vi "ContrastAgent.vi"() -> ()   [LabVIEW 2022 SP3]
uses:
  ViewData/-ReadEye/Header.ctl
  <vilib>/Analysis/5stat.llb/RMS (DBL).vi
  <vilib>/Utility/file.llb/Write Delimited Spreadsheet (string).vi
  <vilib>/Analysis/NI_AALBase.lvlib
  <vilib>/Analysis/NI_AALPro.lvlib
panel:
  in  "Save data":bool
  in  "Header Out":T1={"header info"={"Header"="", "Head length"=0}, "A/D info"={"# rf points per line"=0, "# lines per scan"=0, "sample rate MHz"=0, "# A/D bits"=0, "# bytes per A/D"=0, "TGC Flag"=0, "A/D Type"=""}, "Tranducer Info"={"bandwidth"=0.0, "center freq"=0.0, "start freq"=0.0, "ID"=0}, "Scan Info"={"delay"=0.0, "pivot distance"=0.0, "sector scan angle"=0.0, "operator"="", "Scan Mode"="", "location"=""}, "Time/Date Info"={"date"="", "time"=""}, "RF Info"={"RF file name"="", "RF file att"="", "RF cal file name"="", "RF cal file att"=""}, "Patient Info"={"ID"="", "extended ID"="", "age"=0, "sex"="", "previously\nscanned"="", "PSA"=0.0, "LOS"=1, "Ethnicty 2"=3, "Race"=3}, "Tissue Type"={"organ"=0, "disease type"=0, "disease location"=0, "IQ_pts"=0, "RcvBuffer"=0, "RcvFrame"=0, "IQBuff"=0, "IQFrame"=0, "IQPage"=0}, "Votage scaling"={"Digitizer (dB)"=0.0, "Gain (dB)"=0.0, "Atten (dB)"=0.0}, "Comment"="", "Misc Info"={"avg num"=0, "c speed"=0, "Div By or SF zones"=0, "XMIT CHS"=0, "RCV CHS"=0, "Xmit angle"=0.0}, "Therapy Parameters"={"Theraputic Freq (MHz)"=0.0, "Time on (s)"=0.0, "Therapy amplitude (mV)"=0.0, "Lines Before"=0, "Lines After"=0}, "Scan Settings"={"Energy (uJ or V)"=0, "Damp (Ohm) or Fc"=0, "HP Filt (KHz)"=0, "LP Filt (MHz)"=0, "Gain (db)"=0, "prf (kHz)"=0.0, "Distance between\nscan lines (um)"=0, "Distance between\nscan planes (um)"=0, "Scan line gap (um)"=0.0, "Scan plane gap (um)"=0.0}, "Compression Parameters"={"F1 (MHz)"=0.0, "F2 (MHz)"=0.0, "% taper"=0.0, "duration"=0.0}, "Patient Info Xtra"={"First Name"="", "Last Name"="", "Notes"=""}, "ROI Box"=[0, 0, 0, 0]} {"Compression Parameters"."% taper" min=50 max=1000 format="%.2f"; "Compression Parameters"."F2 (MHz)" format="%.3f"; "Compression Parameters"."F1 (MHz)" format="%.3f"; "Scan Settings"."prf (kHz)" format="%.2f"; "Therapy Parameters"."Therapy amplitude (mV)" min=50 max=1000 format="%.2f"; "Therapy Parameters"."Time on (s)" format="%.3f"; "Therapy Parameters"."Theraputic Freq (MHz)" format="%.3f"; "Patient Info"."Race" items=["Am Ind or Alaska", "Asian", "Hawaiian, Pac Isl", "Black or Afr Amer", "White", "more than one race", "unknown"]; "Patient Info"."Ethnicty 2" items=["Hispanic", "Non-Hispanic", "unknown"]; "Patient Info"."LOS" items=["1", "2", "3", "4", "5"]; "Patient Info"."PSA" format="%.1f"; "Scan Info"."delay" format="%.2f"; "Scan Info"."pivot distance" format="%.2f"; "Scan Info"."sector scan angle" format="%.2f"; "Tranducer Info"."bandwidth" format="%.2f"; "Tranducer Info"."center freq" format="%.2f"; "Tranducer Info"."start freq" format="%.2f"}
  out "match substring":string
  out "noise level":dbl
  out "All Files":string[](array[string])
  out "agent in zone?":bool[](array[boolean])
  out "Array data to save":string[][](array[string])
  out "Numeric":i32
  out "average":sgl[][](array[numeric])
  out "Cts versus start line":i16[](graph)
  in  "How Many":i32
  in  "Sweep":bool
  out "Current file":string
  in  "Use Selected Files":bool
  in  "File Select":i32[](listbox)
  in  "Choose Top":path=path "\\\\vantage-n-wk\\Vantage Data/Adam Doppler/2016-08-12/HFR_03A_20D_08kHz_16MHz_00_EYE"
  in  "image to display":i32 min=0
  in  "start":i32
  out "Total Files":i32
  in  "# of files":i32=2000
  in  "Tab Control":enum32{"Contrast", "Variables"}(tab)
  out "Max dB each image":dbl[](graph)
  out "RF line":dbl[](graph)
  out "Velocity v time 2":dbl[](graph)
  out "Velocity v time":dbl[](graph)
  out "Binary Event Tracking":i16[](graph)
  out "First line":dbl[][](graph)
  out "Raw subset":dbl[][](graph)
  in  "start line":i32=10
  out "Raw data":dbl[][](graph)
  in  "Save  data":bool
  in  "RF Pt start":i32=100
  in  "RF Pts":i32=50
  in  "# rows":i32=17
  out "# drops":i32
  out "RMS noise":T2(graph)
  in  "RMS intervals":i32=10
  out "RMS Noise":dbl
  out "Correlation Shifts":T2(graph)
  in  "Corre Intervals":i32=10
  out "Max Local dB (absolute)":T2(graph)
  in  "Screening":T3={"dB Thresh"=-20.0, "Mask Start"=4, "Mask length"=3}
  out "max dB all":sgl
  out "Velocity":T2(graph)
  in  "Max dB intervals":i32=10
  in  "Vel Intevals":i32=10
  in  "Sub Average":bool
  in  "left rank":i32=2
  in  "dB Threshold":dbl=25.0
  in  "Simple Thresh Count?":bool
  out "Agent?":bool
  in  "fix RMS":dbl format="%0.2f"
  out "# in zone":i16
  in  "fix RMS?":bool
  out "Raw Complex output array":sgl[][][](array[numeric])
  out "Array":sgl[][](array[numeric])
  in  "read?":bool=TRUE
  in  "stop":bool
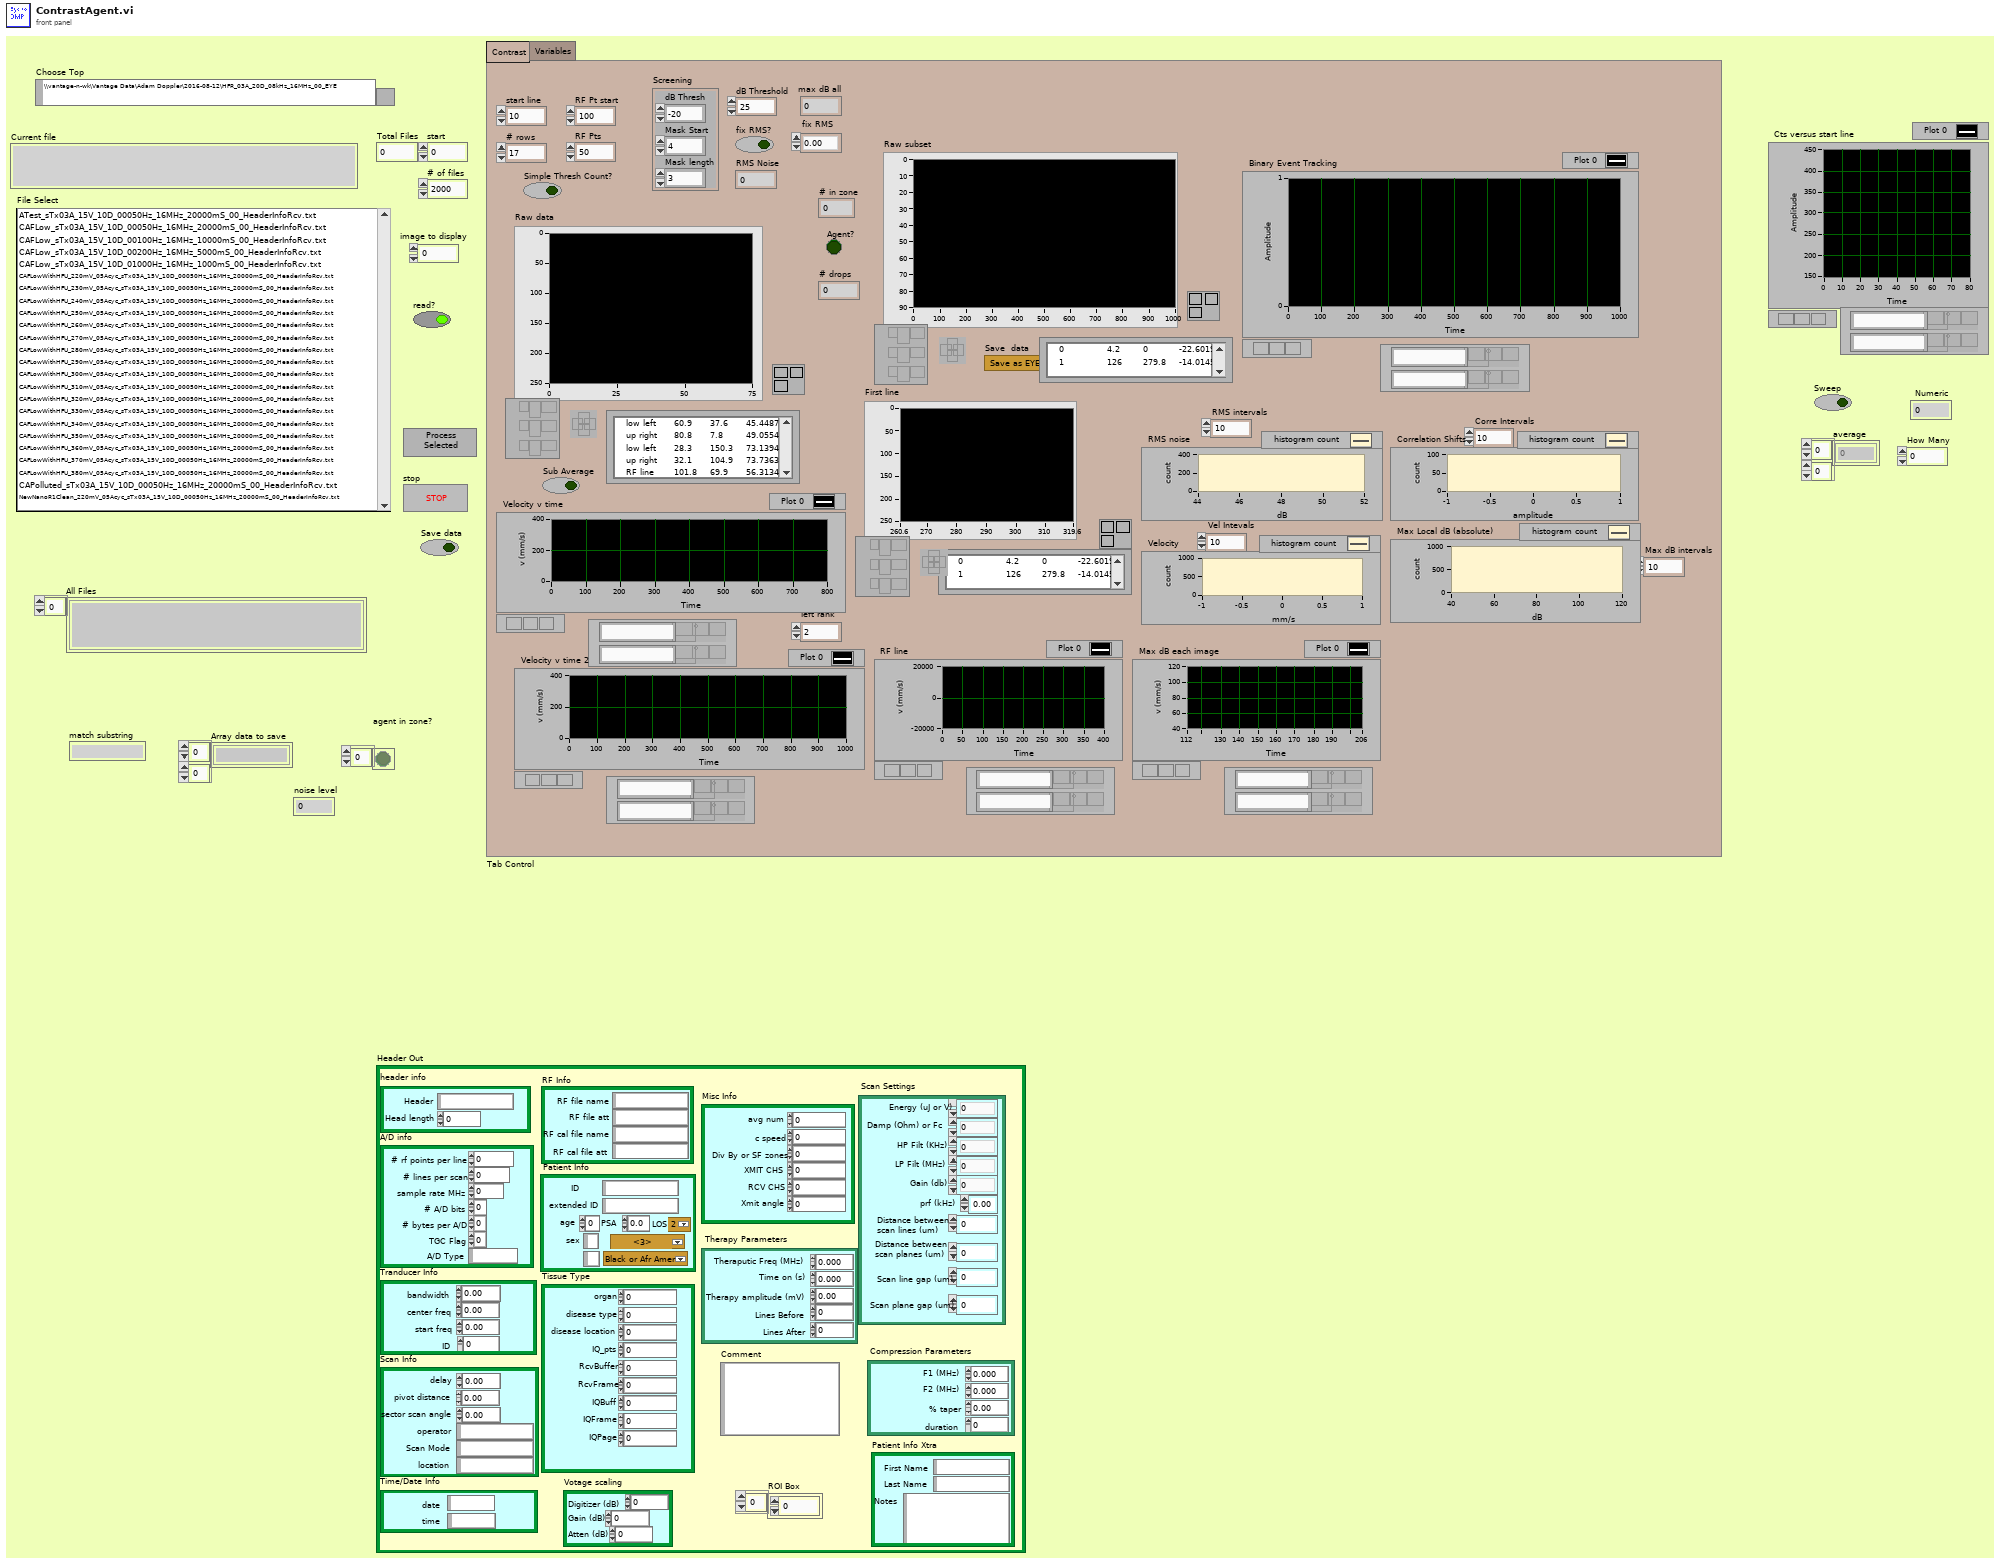
[diagram p1: front panel]
types:
  T1 = typedef "Header.ctl" = cluster{"header info":cluster{"Header":string, "Head length":i16}, "A/D info":cluster{"# rf points per line":u16, "# lines per scan":u16, "sample rate MHz":u16, "# A/D bits":i16, "# bytes per A/D":u16, "TGC Flag":u16, "A/D Type":string}, "Tranducer Info":cluster{"bandwidth":sgl, "center freq":sgl, "start freq":sgl, "ID":i32}, "Scan Info":cluster{"delay":sgl, "pivot distance":sgl, "sector scan angle":sgl, "operator":string, "Scan Mode":string, "location":string}, "Time/Date Info":cluster{"date":string, "time":string}, "RF Info":cluster{"RF file name":string, "RF file att":string, "RF cal file name":string, "RF cal file att":string}, "Patient Info":cluster{"ID":string, "extended ID":string, "age":u16, "sex":string, "previously\nscanned":string, "PSA":sgl, "LOS":u8, "Ethnicty 2":u8, "Race":u8}, "Tissue Type":cluster{"organ":i16, "disease type":i16, "disease location":i16, "IQ_pts":u16, "RcvBuffer":u8, "RcvFrame":u16, "IQBuff":u8, "IQFrame":u16, "IQPage":u8}, "Votage scaling":cluster{"Digitizer (dB)":sgl, "Gain (dB)":sgl, "Atten (dB)":sgl}, "Comment":string, "Misc Info":cluster{"avg num":u16, "c speed":i16, "Div By or SF zones":i16, "XMIT CHS":u8, "RCV CHS":u8, "Xmit angle":sgl}, "Therapy Parameters":cluster{"Theraputic Freq (MHz)":sgl, "Time on (s)":sgl, "Therapy amplitude (mV)":sgl, "Lines Before":u16, "Lines After":u16}, "Scan Settings":cluster{"Energy (uJ or V)":u8, "Damp (Ohm) or Fc":u8, "HP Filt (KHz)":u8, "LP Filt (MHz)":u8, "Gain (db)":u8, "prf (kHz)":sgl, "Distance between\nscan lines (um)":u16, "Distance between\nscan planes (um)":u16, "Scan line gap (um)":sgl, "Scan plane gap (um)":sgl}, "Compression Parameters":cluster{"F1 (MHz)":sgl, "F2 (MHz)":sgl, "% taper":sgl, "duration":sgl}, "Patient Info Xtra":cluster{"First Name":string, "Last Name":string, "Notes":string}, "ROI Box":u16[]}
  T2 = cluster{"X Values":dbl[], "Histogram: h(x)":i32[]}
  T3 = cluster{"dB Thresh":dbl, "Mask Start":i32, "Mask length":i32}
  T4 = enum16{"None", "Raw RF + time stamp", "Save IQAll", "Save IQSum", "Save IQSumReal", "Save Img", "Time Stamps", "unused"}
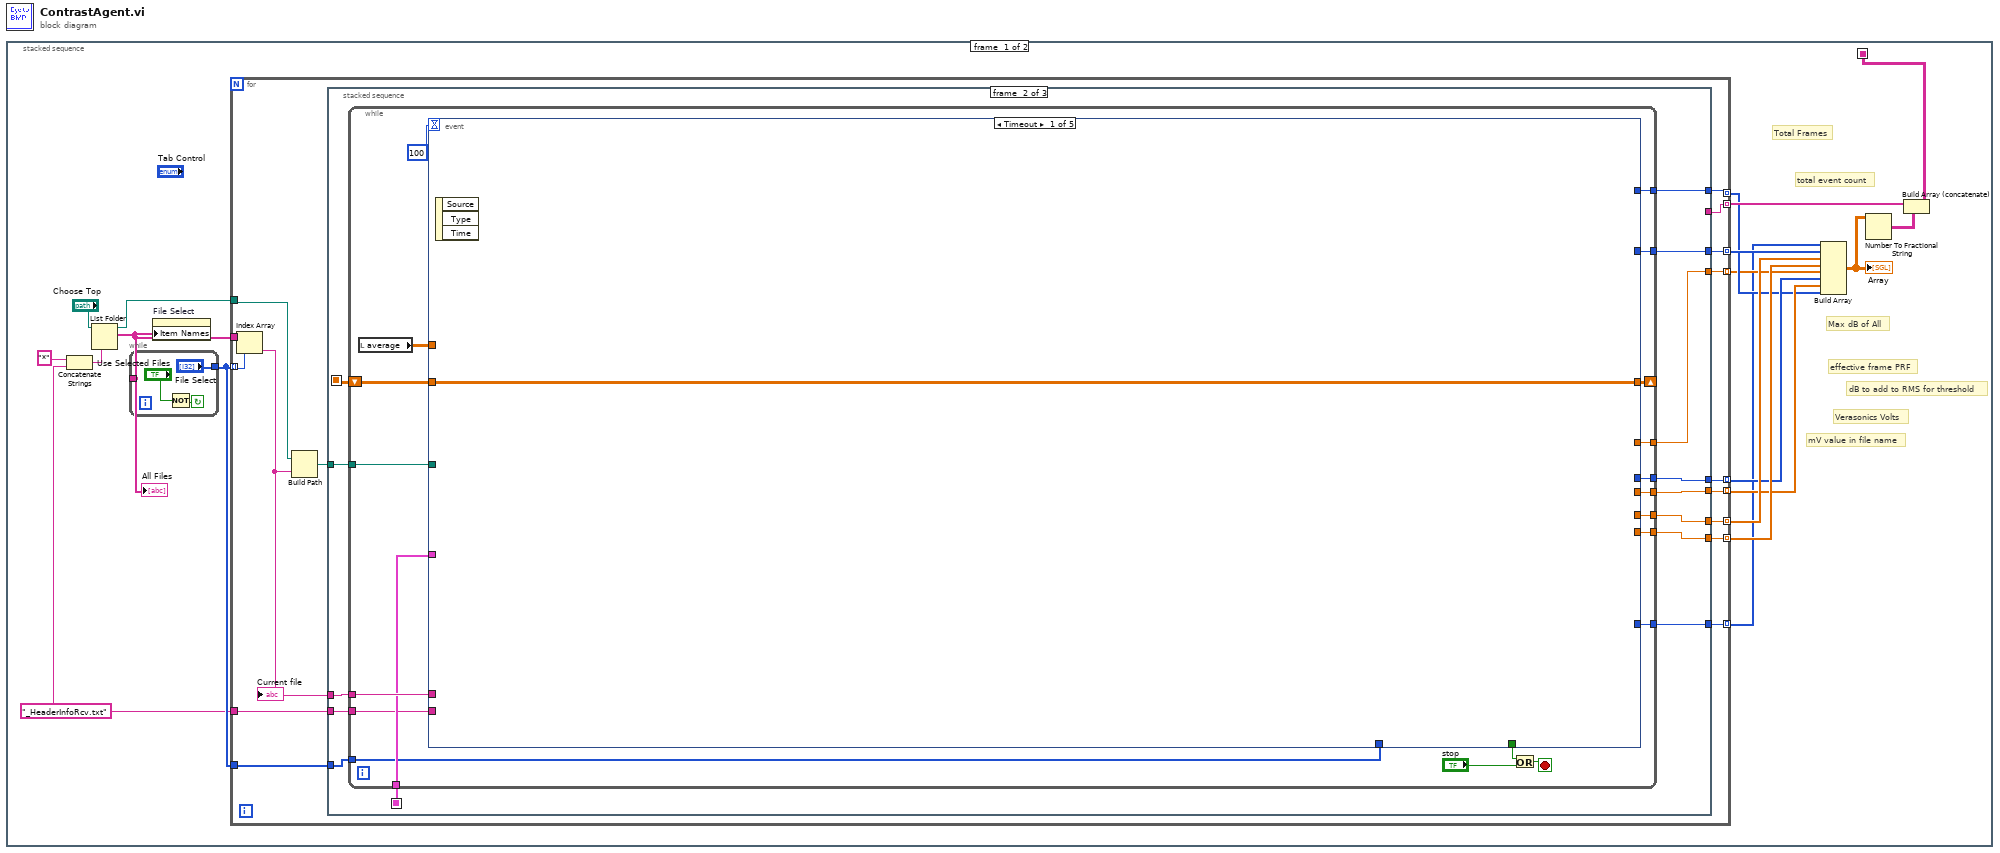
[diagram p0: block diagram]
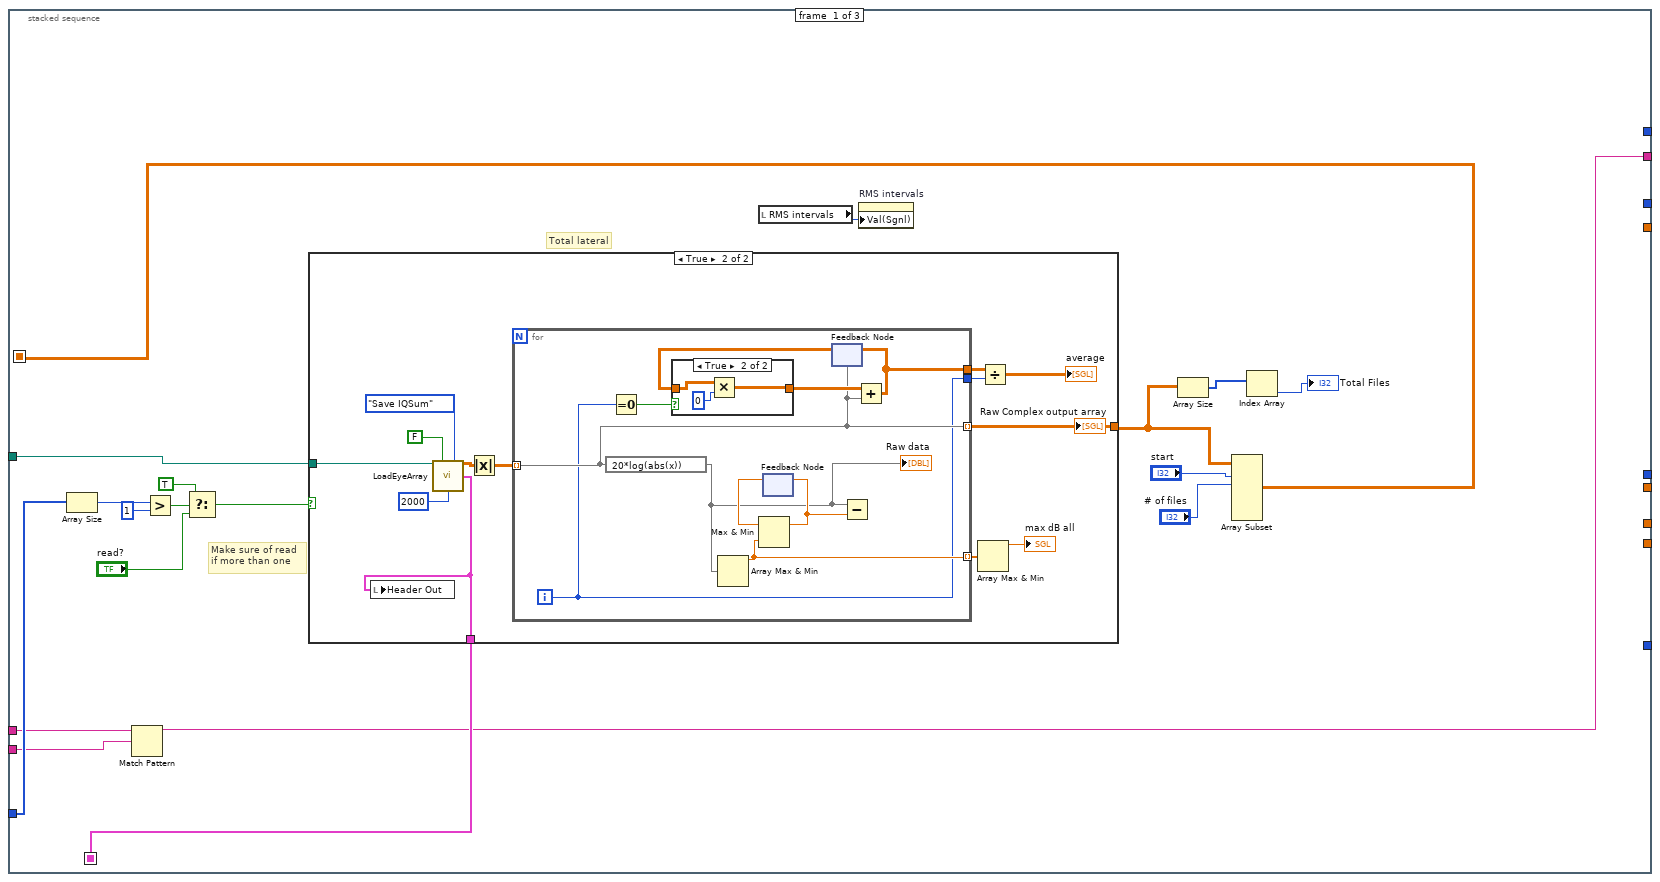
[diagram p2: hidden frame]
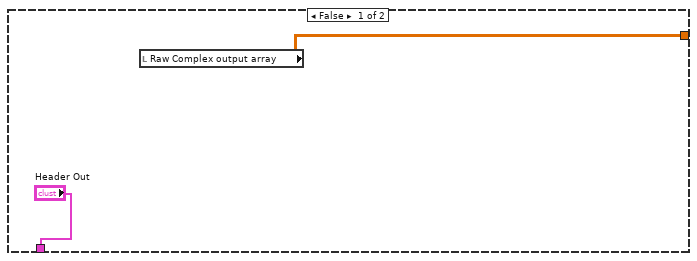
[diagram p3: hidden frame]
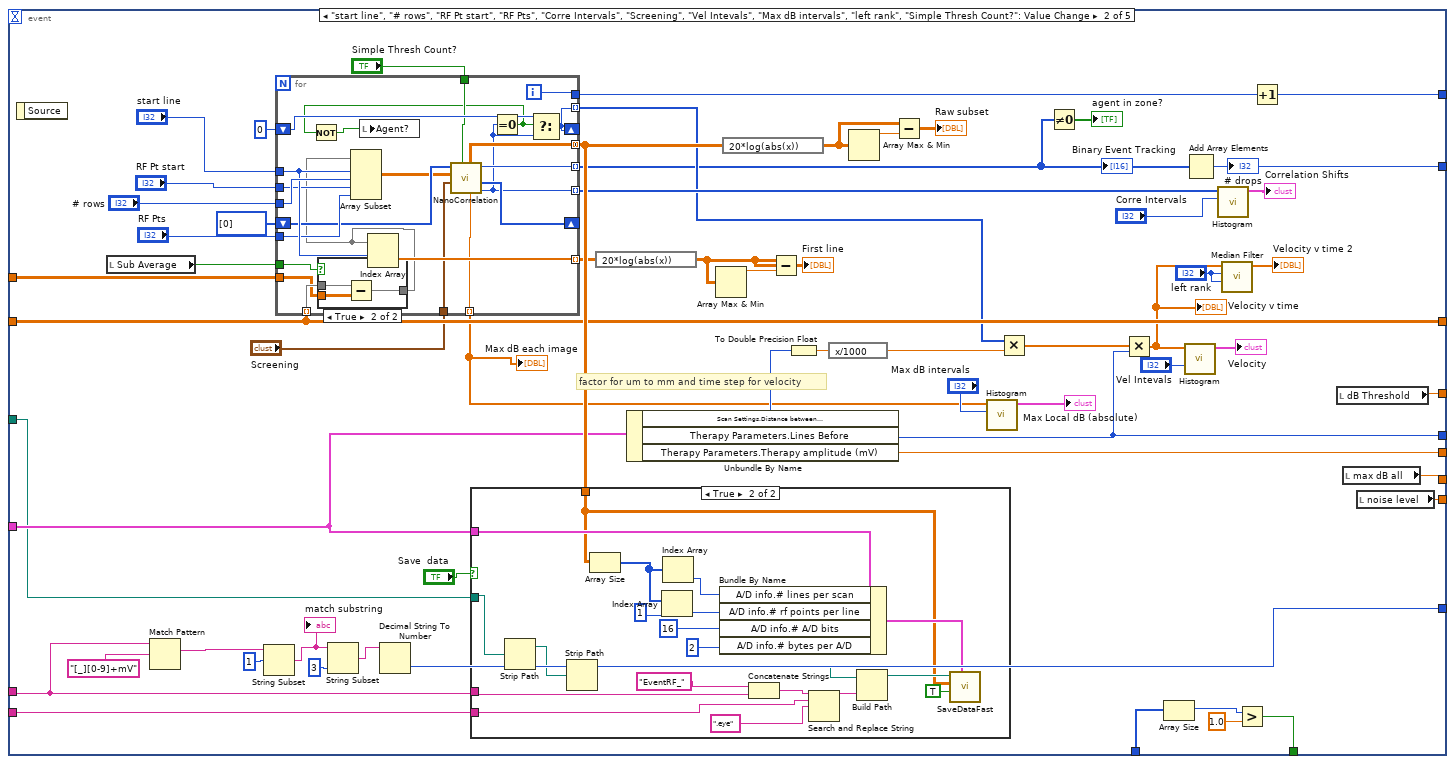
[diagram p5: hidden frame]
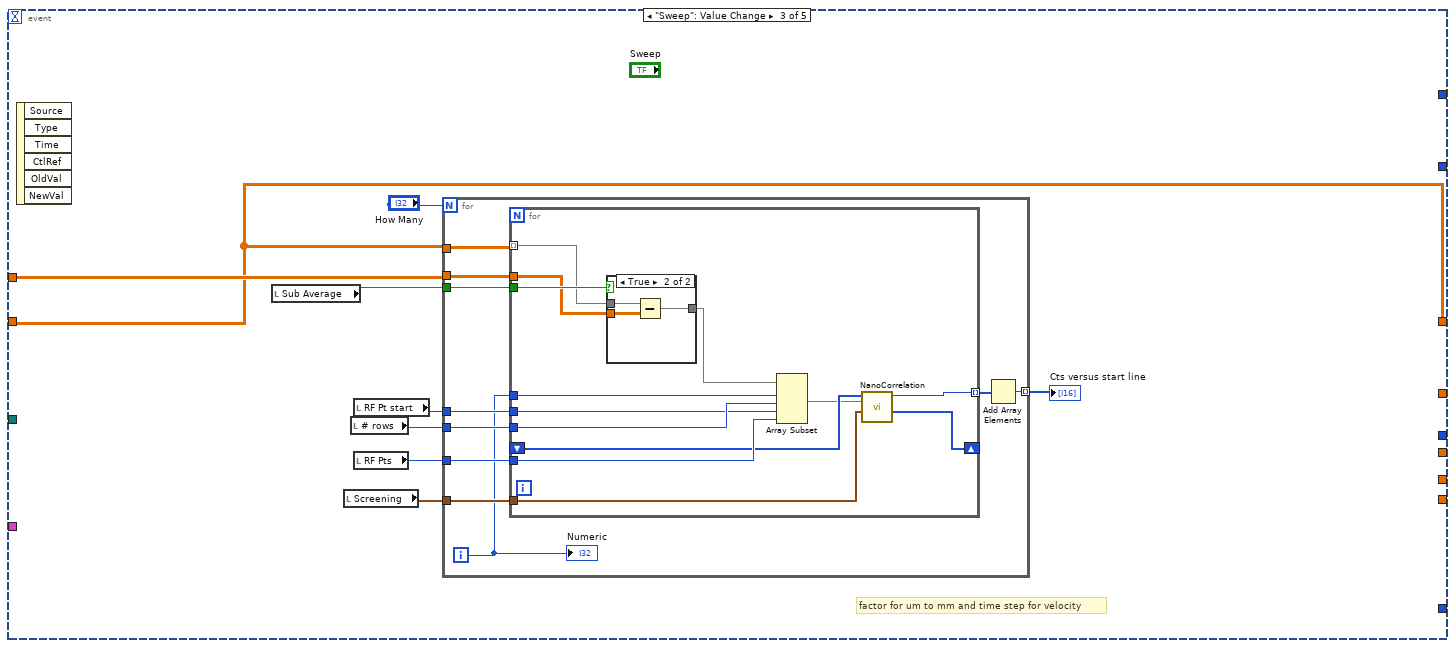
[diagram p8: hidden frame]
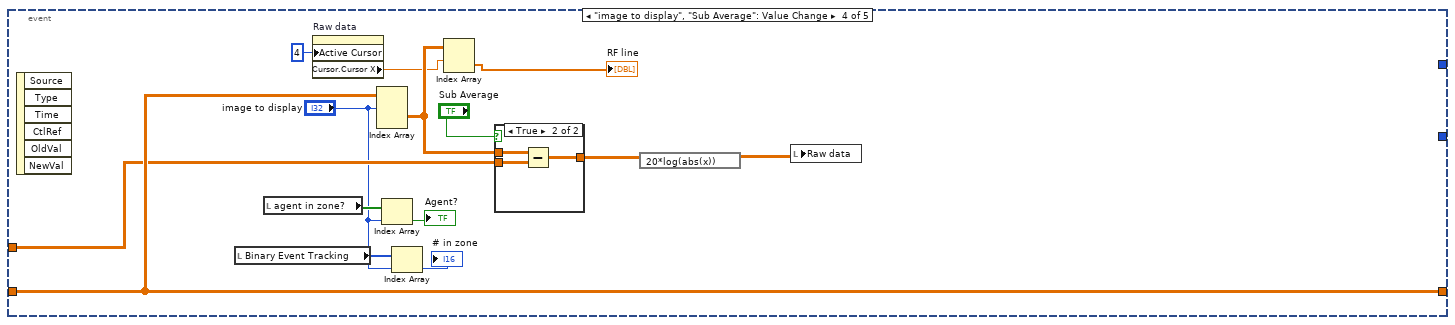
[diagram p10: hidden frame]
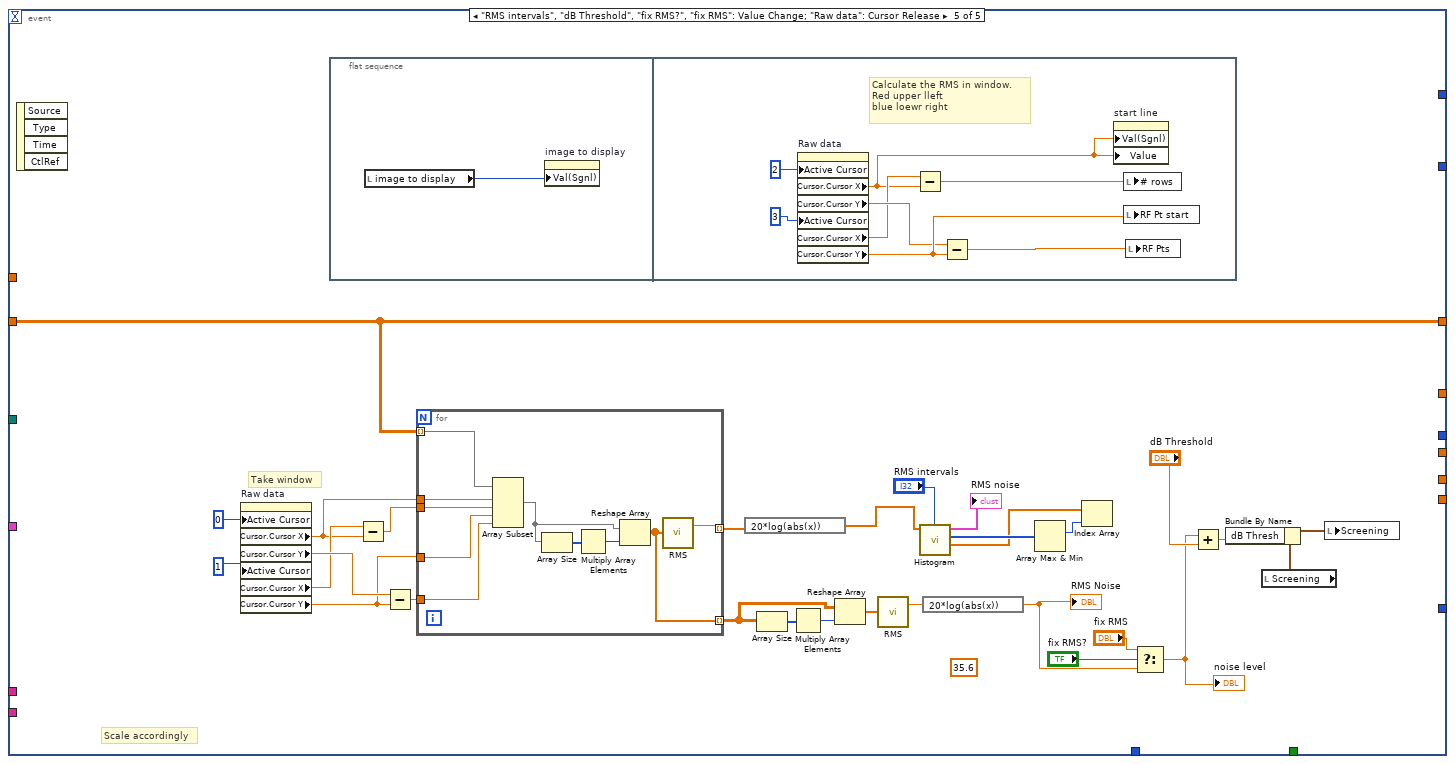
[diagram p12: hidden frame]
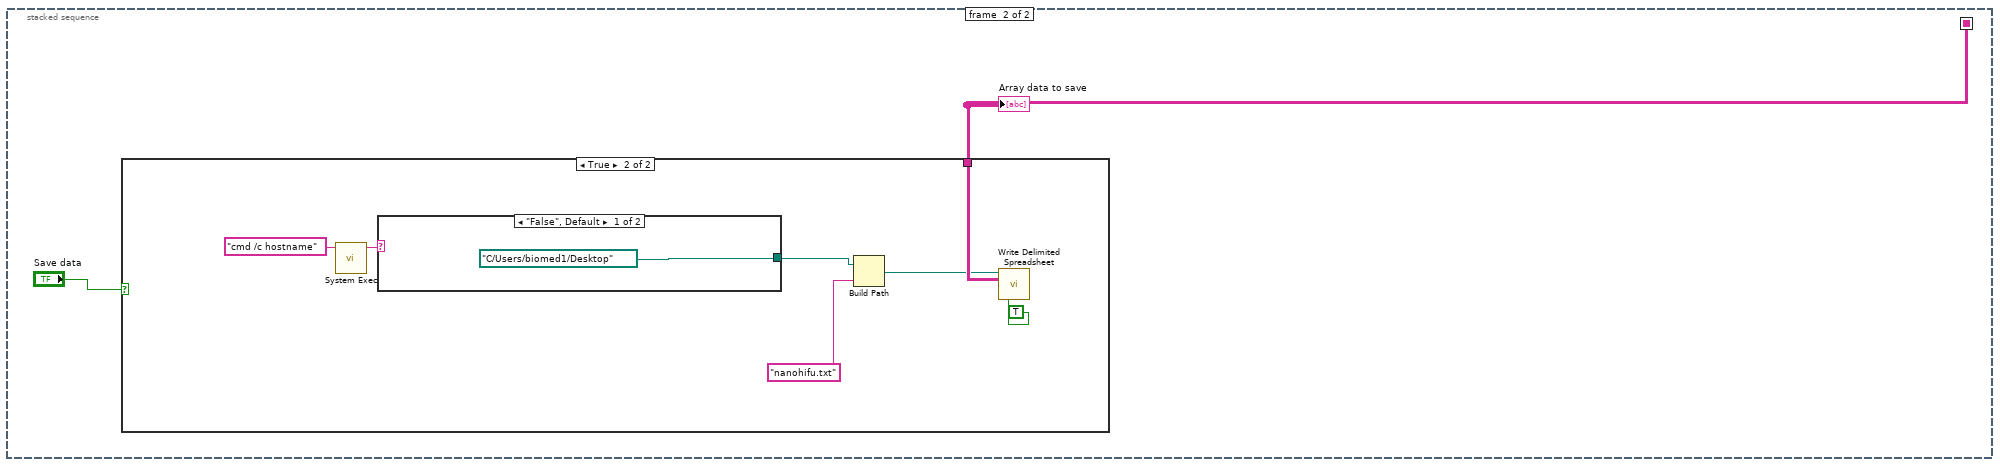
[diagram p14: hidden frame]
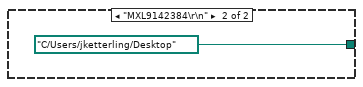
[diagram p16: hidden frame]
diagram:
  n1 = stacked-sequence {
    seq-local: [w5 _] -> [_ w332]
    frame #0 {
      w3 = "_HeaderInfoRcv.txt" ("string")
      # "effective frame PRF"
      # "Total Frames"
      # "Max dB of All"
      # "total event count"
      # "dB to add to RMS for threshold"
      # "mV value in file name"
      # "Verasonics Volts"
      n2 = Concatenate Strings("*" ("file ext"), w3) -> (w1:string)
      n3 = List Folder(path="Choose Top", pattern=w1) -> (path out=w18:path, filenames=w6:string[])  [unwired: 1 in, 3 out]
      "All Files" <- w6
      n4 = while {
        tunnel: ["File Select"] -> w4
        tunnel: w6 -> [_]
        stop <- w22 continue-if-true
        n5 = Not(x="Use Selected Files") -> (.not. x?=w22:bool)
      }
      n6 = property on="File Select" class="LstBox (strict)"("Item Names"=w6) -> ()  [unwired: 2 in, 2 out]
      n7 = for {
        tunnel: w18 -> [w33]
        tunnel: w4 -> [w37] mode=indexing
        tunnel: w6 -> [w38]
        tunnel: [w36] -> w17 mode=indexing
        tunnel: [w35] -> w15 mode=indexing
        tunnel: [w34] -> w16 mode=indexing
        tunnel: [w25] -> w13 mode=indexing
        tunnel: [w31] -> w11 mode=indexing
        tunnel: [w30] -> w10 mode=indexing
        tunnel: [w29] -> w9 mode=indexing
        tunnel: [w28] -> w8 mode=indexing
        tunnel: [w27] -> w7 mode=indexing
        tunnel: w4 -> [w24]
        tunnel: w3 -> [w23]
        n8 = Index Array(array=w38, index=w37) -> (element=w32:string)
        "Current file" <- w32
        n9 = Build Path(base path=w33, name or relative path=w32) -> (appended path=w26:path)
        n10 = stacked-sequence {
          seq-local: [w51 _ _] -> [_ w100 _]
          seq-local: [w55 _ _] -> [_ w90 _]
          tunnel: w32 -> [w41 w99 _]
          tunnel: [_ w98 _] -> w36
          tunnel: [_ w97 _] -> w35
          tunnel: [_ w96 _] -> w34
          tunnel: [_ w95 _] -> w31
          tunnel: [_ w94 _] -> w30
          tunnel: [_ w93 _] -> w29
          tunnel: [_ w92 _] -> w28
          tunnel: [_ w91 _] -> w27
          tunnel: w26 -> [w56 w89 _]
          tunnel: [w39 _ _] -> w25
          tunnel: w24 -> [w48 w88 _]
          tunnel: w23 -> [w40 w87 _]
          frame #0 {
            # "Make sure of read\nif more than one"
            # "Total lateral"
            n11 = Array Size(array=w48) -> (size(s)=w47:i32)
            n12 = Match Pattern(string=w41, regular expression=w40) -> (before substring=w39:string)  [unwired: 1 in, 3 out]
            n13 = Greater?(x=w47, y=1) -> (0:w45:bool)
            n14 = Select(t=TRUE, s=w45, f="read?") -> (s? t:f=w43:bool)
            n15 = case shown="True" w43 {
              tunnel: [w59 w72] -> w52
              tunnel: w56 -> [_ w69]
              tunnel: ["Header Out" w61] -> w55
              frame False {
                n16 = local read "Raw Complex output array"() -> (w59:sgl[][][])
              }
              frame True {
                n17 = call "LoadEyeArray.vi"("directory path of data and header file"=w69, "Split files?"=FALSE, "Type of Read"=T4."Save IQSum", "Cut off"=2000) -> ("RcvBuff 3"=w67:cdb[][][], "Header Out"=w61:T1)  [unwired: 7 in, 3 out]
                n18 = local write "Header Out"(w61) -> ()
                n19 = Absolute Value(x=w67) -> (abs(x)=w66:dbl[][][])
                n20 = for {
                  tunnel: [w75] -> w72 mode=indexing
                  tunnel: [w82] -> w65 mode=indexing
                  tunnel: [w79] -> w64
                  tunnel: w66 -> [w75] mode=indexing
                  tunnel: [w74] -> w63
                  i -> [w74]
                  n21 = expression code="20*log(abs(x))"(w75) -> (w73:dbl[][])
                  "Raw data" <- w73
                  n22 = Equal To 0?(x=w74) -> (x = 0?=w78:bool)
                  n23 = Array Max & Min(array=w73) -> (max value=w82:dbl)  [unwired: 3 out]
                  n24 = feedback #1() -> (w81:dbl)  [unwired: 1 in]
                  n25 = Max & Min(x=w81, y=w82) -> (max(x,y)=w80:dbl)  [unwired: 1 out]
                  n26 = feedback-in #1(w80) -> ()
                  n27 = feedback #2(w75) -> (w76:dbl[][])
                  n28 = case shown="True" w78 {
                    tunnel: [w83 w85] -> w77
                    tunnel: w76 -> [w83 w86]
                    frame False {
                    }
                    frame True {
                      n29 = Multiply(x=w86, y=0) -> (x*y=w85:dbl[][])
                    }
                  }
                  n30 = Subtract(x=w73, y=w80) -> ()  [unwired: 1 out]
                  n31 = Add(x=w77, y=w75) -> (x+y=w79:dbl[][])
                  n32 = feedback-in #2(w79) -> ()
                }
                "Raw Complex output array" <- w72
                n33 = Array Max & Min(array=w65) -> (max value=→"max dB all":dbl)  [unwired: 3 out]
                n34 = Divide(x=w64, y=w63) -> (x/y=→"average":dbl[][])
              }
            }
            n35 = local read "RMS intervals"() -> (w57:i32)
            n36 = property on="RMS intervals" class="DigNum (strict)"("Val(Sgnl)"=w57) -> ()  [unwired: 2 in, 2 out]
            n37 = Array Size(array=w52) -> (size(s)=w54:i32[])
            n38 = Array Subset(array=w52, index (dim 0)="start", length (dim 0)="# of files") -> (w51:dbl[][][])  [unwired: 4 in]
            n39 = Index Array(array=w54) -> (element=→"Total Files":i32)  [unwired: 1 in]
          }
          frame #1 {
            n40 = while {
              tunnel: w99 -> [w119]
              shift-right: [w117] -> _
              shift-left: w100 -> [w120]
              tunnel: [w116] -> w98
              tunnel: [w114] -> w97
              tunnel: [w113] -> w96
              tunnel: [w111] -> w95
              tunnel: [w110] -> w94
              tunnel: [w109] -> w93
              tunnel: [w108] -> w92
              tunnel: [w107] -> w91
              tunnel: w90 -> [w106]
              tunnel: w89 -> [w105]
              tunnel: w88 -> [w103]
              tunnel: w87 -> [w101]
              stop <- w104 stop-if-true
              n41 = local read "average"() -> (w112:sgl[][])
              n42 = event shown="[0] Timeout" {
                selector: _ -> [_ _ _ _ _]
                dyn-events: _ -> [_ _ _ _ _]
                timeout: 100 -> [_ _ _ _ _]
                tunnel: w120 -> [w121 w170 w230 w278 w311]
                tunnel: w119 -> [_ w139 _ _ _]
                tunnel: [w121 w170 w230 w278 w311] -> w117
                tunnel: [_ w158 _ _ _] -> w116
                tunnel: [_ w144 _ _ _] -> w114
                tunnel: [_ w140 _ _ _] -> w113
                tunnel: w112 -> [_ w157 w231 w275 _]
                tunnel: [_ w146 _ _ _] -> w111
                tunnel: [_ w145 _ _ _] -> w110
                tunnel: [_ w142 _ _ _] -> w109
                tunnel: [_ w141 _ _ _] -> w108
                tunnel: [_ w135 _ _ _] -> w107
                tunnel: w106 -> [_ w132 _ _ _]
                tunnel: w105 -> [_ w131 _ _ _]
                tunnel: w103 -> [_ w127 _ _ _]
                tunnel: [_ w125 _ _ _] -> w102
                tunnel: w101 -> [_ w122 _ _ _]
                event Timeout {
                  n43 = event-data() -> ()  [unwired: 1 in, 3 out]
                }
                event "start line", "# rows", "RF Pt start", "RF Pts", "Corre Intervals", "Screening", "Vel Intevals", "Max dB intervals", "left rank", "Simple Thresh Count?": Value Change {
                  # "factor for um to mm and time step for velocity"
                  n44 = event-data() -> ()  [unwired: 1 in, 1 out]
                  n45 = local read "Sub Average"() -> (w152:bool)
                  n46 = Match Pattern(string=w139, regular expression="[_][0-9]+mV") -> (match substring=w130:string)  [unwired: 1 in, 3 out]
                  n47 = String Subset(string=w130, offset (0)=1) -> (substring=w128:string)  [unwired: 1 in]
                  "match substring" <- w128
                  n48 = for {
                    tunnel: w170 -> [w189] mode=indexing
                    tunnel: "start line" -> [w203]
                    tunnel: "# rows" -> [w204]
                    tunnel: [w193] -> w175 mode=concatenating
                    tunnel: [w202] -> w174 mode=indexing
                    tunnel: "RF Pts" -> [w201]
                    tunnel: "RF Pt start" -> [w200]
                    tunnel: [w196] -> w148 mode=indexing
                    shift-right: [w197] -> _
                    shift-left: u8[] [0] ("Agent Indexes") -> [w199]
                    tunnel: [w191] -> w166 mode=indexing
                    tunnel: [w195] -> w133 mode=indexing
                    tunnel: "Screening" -> [w194]
                    tunnel: w157 -> [w188]
                    shift-right: [w190] -> _
                    shift-left: 0 ("max correlation shift") -> [w192]
                    tunnel: [w190] -> w155 mode=indexing
                    tunnel: w152 -> [w186]
                    tunnel: "Simple Thresh Count?" -> [w185]
                    tunnel: [w184] -> w143
                    i -> [w184]
                    n49 = case shown="True" w186 {
                      tunnel: w189 -> [w205 w208]
                      tunnel: [w205 w207] -> w187
                      tunnel: w188 -> [_ w206]
                      frame False {
                      }
                      frame True {
                        n50 = Subtract(x=w208, y=w206) -> (x-y=w207:dbl[][])
                      }
                    }
                    n51 = Array Subset(array=w187, index (row)=w203, length (row)=w204, index (col)=w200, length (col)=w201) -> (w198:dbl[][])
                    n52 = Index Array(array=w187, index (row)=w203) -> (element=w202:dbl[])  [unwired: 1 in]
                    n53 = call "NanoCorrelation.vi"("Simple Thresh Count?"=w185, "Cluster"=w194, "Array"=w198, "Previous Agent Indexes"=w199) -> ("max correlation shift"=w191:i32, "Agent Indexes"=w197:u8[], "New Count"=w196:i16, "Max dB out"=w195:dbl, "RF Trace"=w193:dbl[][])  [unwired: 1 in, 2 out]
                    n54 = Equal To 0?(x=w191) -> (x = 0?=w182:bool)
                    n55 = Not(x=w182) -> (.not. x?=w183:bool)
                    n56 = local write "Agent?"(w183) -> ()
                    n57 = Select(t=w192, s=w182, f=w191) -> (s? t:f=w190:i32)
                  }
                  "Binary Event Tracking" <- w148
                  "Max dB each image" <- w133
                  n58 = String Subset(string=w128, length (rest)=3 ("length (rest)")) -> (substring=w136:string)  [unwired: 1 in]
                  n59 = Decimal String To Number(string=w136) -> (number=w135:i32)  [unwired: 2 in, 1 out]
                  n60 = case shown="True" "Save  data" {
                    tunnel: w132 -> [_ w224]
                    tunnel: w175 -> [_ w219]
                    tunnel: w131 -> [_ w223]
                    tunnel: w139 -> [_ w214]
                    tunnel: w122 -> [_ w209]
                    frame False {
                    }
                    frame True {
                      n61 = Strip Path(path=w223) -> (stripped path=w222:path)  [unwired: 1 out]
                      n62 = Strip Path(path=w222) -> (stripped path=w221:path)  [unwired: 1 out]
                      n63 = Array Size(array=w219) -> (size(s)=w215:i32[])
                      n64 = Index Array(array=w215, index=1) -> (element=w216:i32)
                      n65 = Index Array(array=w215) -> (element=w218:i32)  [unwired: 1 in]
                      n66 = Bundle By Name(cluster=w224, "A/D info.# lines per scan"=w218, "A/D info.# rf points per line"=w216, "A/D info.# A/D bits"=16, "A/D info.# bytes per A/D"=2) -> (w225:T1)
                      n67 = Concatenate Strings("EventRF_" ("string"), w214) -> (w210:string)
                      n68 = Search and Replace String(input string=w210, search string=w209, replace string=".eye" ("string")) -> (result string=w213:string)  [unwired: 5 in, 3 out]
                      n69 = Build Path(base path=w221, name or relative path=w213) -> (appended path=w226:path)
                      n70 = call "SaveDataFast.vi"("Header In"=w225, "Save?"=TRUE, "Data Array"=w219, "File Name and Path"=w226) -> ()  [unwired: 7 in, 1 out]
                    }
                  }
                  n71 = expression code="20*log(abs(x))"(w174) -> (w134:dbl[][])
                  "First line" <- w134
                  n72 = Unbundle By Name(w132) -> ("Scan Settings.Distance between\nscan lines (um)"=w161:u16, "Therapy Parameters.Lines Before"=w146:u16, "Therapy Parameters.Therapy amplitude (mV)"=w145:sgl)
                  n73 = Array Max & Min(array=w134) -> (max value=w173:dbl)  [unwired: 3 out]
                  n74 = expression code="20*log(abs(x))"(w175) -> (w180:dbl[][])
                  n75 = Subtract(x=w134, y=w173) -> ()  [unwired: 1 out]
                  n76 = To Double Precision Float(number=w161) -> (double precision float=w160:dbl)
                  n77 = expression code="x/1000"(w160) -> (w159:dbl)
                  n78 = Array Max & Min(array=w180) -> (max value=w181:dbl)  [unwired: 3 out]
                  n79 = Subtract(x=w180, y=w181) -> (x-y=→"Raw subset":dbl[][])
                  n80 = call <vilib>:"Histogram.vi"("intervals"="Max dB intervals", "X"=w133) -> ("Histogram Graph"=→"Max Local dB (absolute)":T2)  [unwired: 6 in, 3 out]
                  n81 = Multiply(x=w155, y=w159) -> (x*y=w165:dbl[])
                  n82 = Not Equal To 0?(x=w148) -> (x != 0?=→"agent in zone?":bool[])
                  n83 = Multiply(x=w165, y=w146) -> (x*y=w153:dbl[])
                  "Velocity v time" <- w153
                  n84 = Array Size(array=w127) -> (size(s)=w124:i32)
                  n85 = call <vilib>:"Histogram.vi"("intervals"="Vel Intevals", "X"=w153) -> ("Histogram Graph"=→"Velocity":T2)  [unwired: 6 in, 3 out]
                  n86 = Add Array Elements(numeric array=w148) -> (sum=w158:i16)
                  "# drops" <- w158
                  n87 = call <vilib>:"Histogram.vi"("intervals"="Corre Intervals", "X"=w166) -> ("Histogram Graph"=→"Correlation Shifts":T2)  [unwired: 6 in, 3 out]
                  n88 = call <vilib>:"Median Filter.vi"("right rank"="left rank", "left rank"="left rank", "X"=w153) -> ("Filtered X"=→"Velocity v time 2":dbl[])  [unwired: 7 in, 1 out]
                  n89 = Greater?(x=w124, y=1.0) -> (0:w125:bool)
                  n90 = Increment(x=w143) -> (x+1=w142:i32)
                  n91 = local read "dB Threshold"() -> (w141:dbl)
                  n92 = local read "max dB all"() -> (w140:sgl)
                  n93 = local read "noise level"() -> (w144:dbl)
                }
                event "Sweep": Value Change {
                  # "factor for um to mm and time step for velocity"
                  n94 = event-data() -> ()  [unwired: 1 in, 6 out]
                  n95 = local read "Sub Average"() -> (w229:bool)
                  n96 = local read "Screening"() -> (w234:T3)
                  n97 = local read "# rows"() -> (w236:i32)
                  n98 = local read "RF Pt start"() -> (w237:i32)
                  n99 = local read "RF Pts"() -> (w235:i32)
                  n100 = for {
                    N: "How Many" -> [_]
                    tunnel: w230 -> [w247]
                    tunnel: w237 -> [w246]
                    tunnel: w236 -> [w245]
                    tunnel: w235 -> [w244]
                    tunnel: w234 -> [w243]
                    tunnel: [w241] -> w232 mode=indexing
                    tunnel: w231 -> [w239]
                    tunnel: w229 -> [w238]
                    i -> [w240]
                    n101 = for {
                      tunnel: w245 -> [w260]
                      tunnel: w244 -> [w259]
                      tunnel: w246 -> [w258]
                      tunnel: [w255] -> w242 mode=indexing
                      shift-right: [w256] -> _
                      shift-left: _ -> [w257]
                      tunnel: w243 -> [w254]
                      tunnel: w247 -> [w249] mode=indexing
                      tunnel: w240 -> [w253]
                      tunnel: w239 -> [w250]
                      tunnel: w238 -> [w251]
                      n102 = case shown="True" w251 {
                        tunnel: w249 -> [w261 w264]
                        tunnel: [w261 w263] -> w248
                        tunnel: w250 -> [_ w262]
                        frame False {
                        }
                        frame True {
                          n103 = Subtract(x=w264, y=w262) -> (x-y=w263:dbl[][])
                        }
                      }
                      n104 = Array Subset(array=w248, index (row)=w253, length (row)=w260, index (col)=w258, length (col)=w259) -> (w252:dbl[][])
                      n105 = call "NanoCorrelation.vi"("Cluster"=w254, "Array"=w252, "Previous Agent Indexes"=w257) -> ("Agent Indexes"=w256:u8[], "New Count"=w255:i16)  [unwired: 2 in, 5 out]
                    }
                    n106 = Add Array Elements(numeric array=w242) -> (sum=w241:i16)
                    "Numeric" <- w240
                  }
                  "Cts versus start line" <- w232
                }
                event "image to display", "Sub Average": Value Change {
                  n107 = event-data() -> ()  [unwired: 1 in, 6 out]
                  n108 = local read "Binary Event Tracking"() -> (w267:i16[])
                  n109 = local read "agent in zone?"() -> (w274:bool[])
                  n110 = property on="Raw data" class="IntGraph (strict)"("Active Cursor"=u32 4) -> ("Cursor.Cursor X"=w270:dbl)  [unwired: 2 in, 2 out]
                  n111 = Index Array(array=w278, index (dim 0)="image to display") -> (element=w271:dbl[][])  [unwired: 2 in]
                  n112 = Index Array(array=w274, index="image to display") -> (element=→"Agent?":bool)
                  n113 = Index Array(array=w267, index="image to display") -> (element=→"# in zone":i16)
                  n114 = Index Array(array=w271, index (row)=w270) -> (element=→"RF line":dbl[])  [unwired: 1 in]
                  n115 = case shown="True" "Sub Average" {
                    tunnel: w271 -> [w279 w282]
                    tunnel: [w279 w281] -> w277
                    tunnel: w275 -> [_ w280]
                    frame False {
                    }
                    frame True {
                      n116 = Subtract(x=w282, y=w280) -> (x-y=w281:dbl[][])
                    }
                  }
                  n117 = expression code="20*log(abs(x))"(w277) -> (w268:dbl[][])
                  n118 = local write "Raw data"(w268) -> ()
                }
                event "RMS intervals", "dB Threshold", "fix RMS?", "fix RMS": Value Change; "Raw data": Cursor Release {
                  (unwired) 35.6
                  # "Take window"
                  # "Scale accordingly"
                  n119 = event-data() -> ()  [unwired: 1 in, 4 out]
                  n120 = property on="Raw data" class="IntGraph (strict)"("Active Cursor"=u32 0 ("Write Attribute"), "Active Cursor"=u32 1 ("Write Attribute")) -> ("Cursor.Cursor X"=w301:dbl, "Cursor.Cursor Y"=w303:dbl, "Cursor.Cursor X"=w302:dbl, "Cursor.Cursor Y"=w298:dbl)  [unwired: 2 in, 2 out]
                  n121 = flat-sequence {
                    frame #0 {
                      n122 = local read "image to display"() -> (w312:i32)
                      n123 = property on="image to display" class="DigNum (strict)"("Val(Sgnl)"=w312) -> ()  [unwired: 2 in, 2 out]
                    }
                    frame #1 {
                      # "Calculate the RMS in window.\nRed upper lleft\nblue loewr right"
                      n124 = property on="Raw data" class="IntGraph (strict)"("Active Cursor"=u32 2 ("Write Attribute"), "Active Cursor"=u32 3 ("Write Attribute")) -> ("Cursor.Cursor X"=w315:dbl, "Cursor.Cursor Y"=w317:dbl, "Cursor.Cursor X"=w316:dbl, "Cursor.Cursor Y"=w318:dbl)  [unwired: 2 in, 2 out]
                      n125 = Subtract(x=w316, y=w315) -> (x-y=w320:dbl)
                      n126 = Subtract(x=w317, y=w318) -> (x-y=w319:dbl)
                      n127 = property on="start line" class="DigNum (strict)"("Val(Sgnl)"=w315, "Value"=w315) -> ()  [unwired: 2 in, 2 out]
                      n128 = local write "# rows"(w320) -> ()
                      n129 = local write "RF Pt start"(w318) -> ()
                      n130 = local write "RF Pts"(w319) -> ()
                    }
                  }
                  n131 = Subtract(x=w302, y=w301) -> (x-y=w300:dbl)
                  n132 = Subtract(x=w303, y=w298) -> (x-y=w299:dbl)
                  n133 = for {
                    tunnel: w311 -> [w327] mode=indexing
                    tunnel: [w322] -> w295 mode=indexing
                    tunnel: w301 -> [w326]
                    tunnel: w300 -> [w325]
                    tunnel: w299 -> [w324]
                    tunnel: w298 -> [w323]
                    tunnel: [w321] -> w290 mode=indexing
                    n134 = Array Subset(array=w327, index (row)=w326, length (row)=w325, index (col)=w323, length (col)=w324) -> (w328:dbl[][])
                    n135 = Array Size(array=w328) -> (size(s)=w330:i32[])
                    n136 = Multiply Array Elements(1:w330) -> (0:w329:i32)
                    n137 = Reshape Array(w328, w329) -> (w321:dbl[])
                    n138 = call-poly <vilib>:"RMS.vi"("X"=w321) -> ("rms value"=w322:dbl)  [unwired: 1 out]
                  }
                  n139 = expression code="20*log(abs(x))"(w295) -> (w288:dbl[])
                  n140 = Array Size(array=w290) -> (size(s)=w293:i32[])
                  n141 = Multiply Array Elements(1:w293) -> (0:w291:i32)
                  n142 = Reshape Array(w290, w291) -> (w292:dbl[])
                  n143 = call-poly <vilib>:"RMS.vi"("X"=w292) -> ("rms value"=w289:dbl)  [unwired: 1 out]
                  n144 = call <vilib>:"Histogram.vi"("intervals"="RMS intervals", "X"=w288) -> ("X Values"=w306:dbl[], "Histogram: h(x)"=w307:i32[], "Histogram Graph"=→"RMS noise":T2)  [unwired: 6 in, 1 out]
                  n145 = expression code="20*log(abs(x))"(w289) -> (w284:dbl)
                  "RMS Noise" <- w284
                  n146 = Array Max & Min(array=w307) -> (max index (indices)=w308:i32)  [unwired: 3 out]
                  n147 = Index Array(array=w306, index=w308) -> ()  [unwired: 1 out]
                  n148 = Select(t="fix RMS", s="fix RMS?", f=w284) -> (s? t:f=w286:dbl)
                  "noise level" <- w286
                  n149 = Add(x=w286, y="dB Threshold") -> (x+y=w287:dbl)
                  n150 = local read "Screening"() -> (w297:T3)
                  n151 = Bundle By Name(cluster=w297, "dB Thresh"=w287) -> (w296:T3)
                  n152 = local write "Screening"(w296) -> ()
                }
              }
              n153 = Or(x=w102, y="stop") -> (x .or. y?=w104:bool)
            }
          }
          frame #2 {
          }
        }
      }
      n154 = Build Array(w7, w17, w16, w15, w8, w11, w10, w9) -> (w14:dbl[][])
      "Array" <- w14
      n155 = Number To Fractional String(number=w14) -> (F-format string=w12:string[][])  [unwired: 3 in]
      n156 = Build Array (concatenate)(w13, w12) -> (w5:string[][])
    }
    frame #1 {
      n157 = case shown="True" "Save data" {
        tunnel: w332 -> [_ w336]
        frame False {
        }
        frame True {
          n158 = call <vilib>:"System Exec.vi"("command line"="cmd /c hostname") -> ("standard output"=w338:string)  [unwired: 7 in, 3 out]
          n159 = case shown="\"False\", Default" w338 {
            tunnel: [path "C:/Users/biomed1/Desktop" ("file path (dialog if empty)") path "C:/Users/jketterling/Desktop" ("file path (dialog if empty)")] -> w335
            frame "False", Default {
            }
            frame "MXL9142384\r\n" {
            }
          }
          n160 = Build Path(base path=w335, name or relative path="nanohifu.txt") -> (appended path=w333:path)
          n161 = call-poly <vilib>:"Write Delimited Spreadsheet.vi"("file path (dialog if empty)"=w333, "2D data"=w336, "transpose? (no:F)"=TRUE) -> ()  [unwired: 11 in, 2 out]
        }
      }
      "Array data to save" <- w332
    }
  }
